vi "State Control.vi"(8 "Error Input":errorcluster, 10 "Input States":T1=enum."Exit", 11 "Stop":bool) -> (2 "Output State":T1)   [LabVIEW 2015]
uses:
  State Enum.ctl
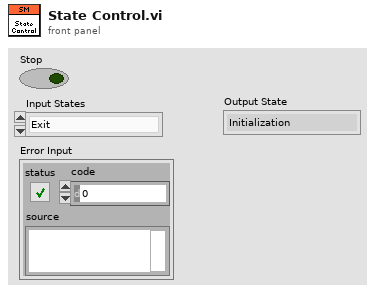
[diagram p1: front panel]
types:
  T1 = typedef "State Enum.ctl" = enum16{"Initialization", "Wait", "Update Controller Info", "Update Reference Info", "Update Detector Trigger Info", "Update Datalog Info", "Check FPGA Status", "Reading FIFO", "Exit"}
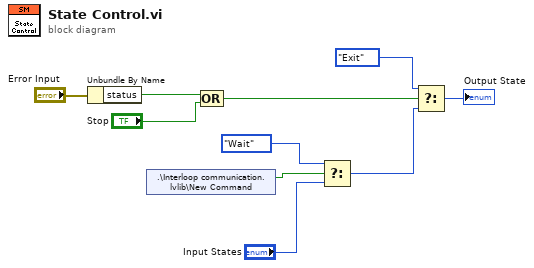
[diagram p0: block diagram]
diagram:
  n1 = Unbundle By Name "Unbundle By Name"("Error Input") -> ("status"=w9:bool)
  n2 = shared-variable ".\\Interloop communication.lvlib\\New Command"() -> (w4:bool)  [unwired: 1 in, 1 out]
  n3 = Compound Arithmetic op=OR(w9, "Stop") -> (w7:bool)
  n4 = Select(t=State_Enum."Wait", s=w4, f="Input States") -> (s? t:f=w2:T1)
  n5 = Select(t=State_Enum."Exit" ("States"), s=w7, f=w2) -> (s? t:f=→"Output State":T1)
